vi "Test SUBACK packet.vi"(8 "error in (no error)":errorcluster) -> (0 "error out":errorcluster)   [LabVIEW 2013]
uses:
  source/Control Packets/SUBACK/Subscription Success Code.ctl
  source/Control Packets/ControlPacket/QualityOfService -- enum.ctl
  source/Control Packets/SUBACK/SUBACK.lvclass
  source/Control Packets/ControlPacket/ControlPacket.lvclass/ControlPacket.ctl
  source/Control Packets/ControlPacket/ControlPacket.lvclass
  <vilib>/addons/_JKI Toolkits/Caraya/classes/Test/Test.lvclass
  <vilib>/addons/_JKI Toolkits/Caraya/classes/Assert/Assert.lvclass
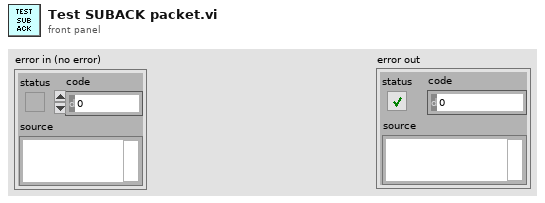
[diagram p1: front panel]
types:
  T1 = typedef "MQTT_Control_Packets.lvlib/SUBACK.lvclass/Subscription Success Code.ctl" = cluster{"Subscription Failure":bool, "QoS":T2}
  T2 = typedef "MQTT_Control_Packets.lvlib/ControlPacket.lvclass/QualityOfService -- enum.ctl" = enum16{"0 (At Most Once)", "1 (At Least Once)", "2 (Exactly Once)"}
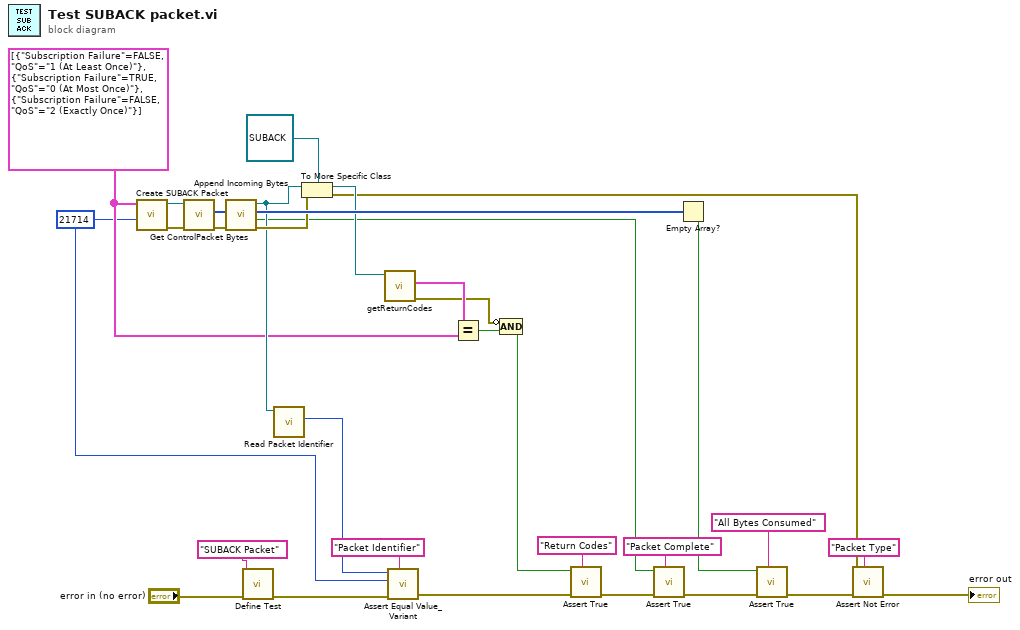
[diagram p0: block diagram]
diagram:
  w23 = T1[] [{"Subscription Failure"=FALSE, "QoS"=enum."1 (At Least Once)"}, {"Subscription Failure"=TRUE, "QoS"=enum."0 (At Most Once)"}, {"Subscription Failure"=FALSE, "QoS"=enum."2 (Exactly Once)"}] ("Return Codes")
  w9 = u16 21714 ("Packet ID")
  n1 = call "Create SUBACK Packet.vi"("Packet ID"=w9, "Return Codes"=w23) -> ("error out"=w27:errorcluster, "SUBACK"=w26:refnum<class "SUBACK.lvclass">)  [unwired: 8 in]
  n2 = call "Get ControlPacket Bytes.vi"("error in (no error)"=w27, "ControlPacket"=w26) -> ("error out"=w30:errorcluster, "Bytes Stream"=w32:u8[])  [unwired: 6 in, 2 out]
  n3 = call "Append Incoming Bytes.vi"("error in (no error)"=w30, "Incoming Packets"=w32) -> ("error out"=w29:errorcluster, "Complete Packet"=w5:bool, "Remaining Packets"=w31:u8[], "ControlPacket"=w28:refnum<class "ControlPacket.lvclass">)  [unwired: 6 in]
  n4 = call <vilib>:"Define Test.vi"("error in (no error)"="error in (no error)", "Label (VI Title)"="SUBACK Packet") -> ("error out"=w14:errorcluster)  [unwired: 9 in]
  n5 = call "Read Packet Identifier.vi"("ControlPacket in"=w28) -> ("Packet Identifier"=w10:u16)  [unwired: 9 in, 1 out]
  n6 = To More Specific Class(target class=refnum<class "SUBACK.lvclass"> refnum ("MQTT_Control_Packets.lvlib:SUBACK.lvclass"), reference=w28, error in=w29) -> (specific class reference=w25:refnum<class "SUBACK.lvclass">, error out=w7:errorcluster)
  n7 = call "getReturnCodes.vi"("SUBACK in"=w25) -> ("error out"=w21:errorcluster, "Subscription Success"=w24:T1[])  [unwired: 8 in, 1 out]
  n8 = call <vilib>:"Assert Equal Value_Variant.vi"("Label"="Packet Identifier" ("Label (VI Title)"), "error in (no error)"=w14, "Y"=w9, "X"=w10) -> ("error out"=w3:errorcluster)  [unwired: 7 in]
  n9 = Equal?(x=w24, y=w23) -> (x = y?=w22:bool)
  n10 = Compound Arithmetic op=AND(invert w21, w22) -> (w1:bool)
  n11 = call <vilib>:"Assert True.vi"("Label"="Return Codes" ("Label (VI Title)"), "error in (no error)"=w3, "True?"=w1) -> ("error out"=w2:errorcluster)  [unwired: 8 in]
  n12 = call <vilib>:"Assert True.vi"("Label"="Packet Complete" ("Label (VI Title)"), "error in (no error)"=w2, "True?"=w5) -> ("error out"=w15:errorcluster)  [unwired: 8 in]
  n13 = Empty Array?(array=w31) -> (empty?=w6:bool)
  n14 = call <vilib>:"Assert True.vi"("Label"="All Bytes Consumed" ("Label (VI Title)"), "error in (no error)"=w15, "True?"=w6) -> ("error out"=w11:errorcluster)  [unwired: 8 in]
  n15 = call <vilib>:"Assert Not Error.vi"("Label"="Packet Type" ("Label (VI Title)"), "error in (no error)"=w11, "Not Error?"=w7) -> ("error out"=→"error out":errorcluster)  [unwired: 8 in]
